vi "memory_load_C_1.vi"() -> ()   [LabVIEW 2020]
panel:
  out "Array":fxp<+/-,32,16>[](array[numeric])
  out "Init Data Out":fxp<+/-,32,16>[][](array[numeric])
  out "size(s)":i32
  # "For Initialization VI requirements and help, please read directions located on Block Diagram."
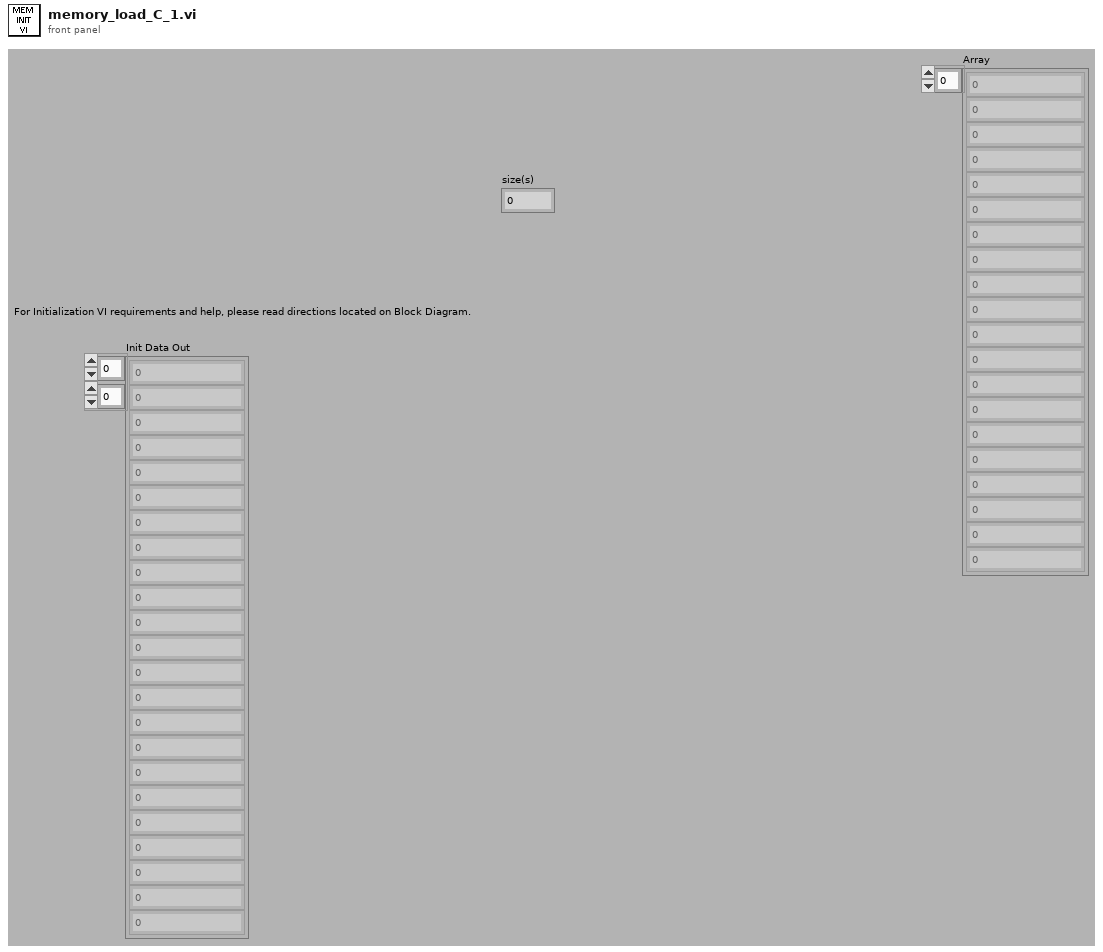
[diagram p1: front panel]
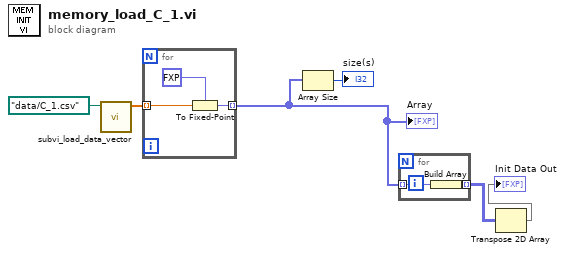
[diagram p0: block diagram]
diagram:
  n1 = call "subvi_load_data_vector.vi"("default name"=path "data/C_1.csv") -> ("array type (2D Dbl) out"=w5:dbl[])  [unwired: 10 in]
  n2 = for {
    tunnel: w5 -> [w9] mode=indexing
    tunnel: [w8] -> w3 mode=indexing
    n3 = To Fixed-Point(fixed-point type=fxp<+/-,32,16> 0.0 ("fixed-point"), number=w9) -> (fixed-point=w8:fxp<+/-,32,16>)
  }
  "Array" <- w3
  n4 = Array Size(array=w3) -> (size(s)=→"size(s)":i32)
  n5 = for {
    tunnel: w3 -> [w11] mode=indexing
    tunnel: [w10] -> w2 mode=indexing
    n6 = Build Array(w11) -> (w10:fxp<+/-,32,16>[])
  }
  n7 = Transpose 2D Array(2D array=w2) -> (transposed array=→"Init Data Out":fxp<+/-,32,16>[][])
